vi "Destroy Queues.vi"(8 "error in (no error)":errorcluster) -> (0 "error out":errorcluster)   [LabVIEW 2017]
uses:
  Reference Action.ctl
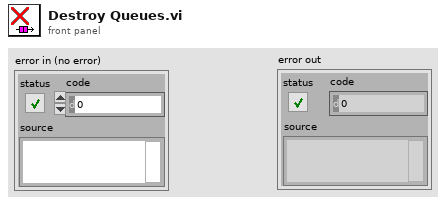
[diagram p1: front panel]
types:
  T1 = typedef "Reference Action.ctl" = enum16{"Set", "Get"}
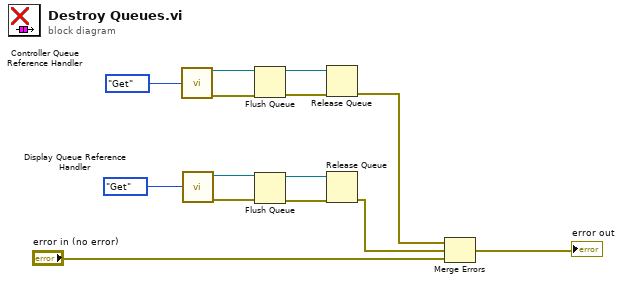
[diagram p0: block diagram]
diagram:
  n1 = call "Controller Queue Reference Handler.vi"("Reference Action"=Reference_Action."Get") -> ("Error Out"=w14:errorcluster, "Queue Ref Out"=w12:refnum<queue>)  [unwired: 9 in]
  n2 = call "Display Queue Reference Handler.vi"("Reference Action"=Reference_Action."Get") -> ("Error Out"=w8:errorcluster, "Queue Ref Out"=w7:refnum<queue>)  [unwired: 9 in]
  n3 = Flush Queue(queue=w12, error in (no error)=w14) -> (queue out=w6:refnum<queue>, error out=w13:errorcluster)  [unwired: 1 out]
  n4 = Flush Queue(queue=w7, error in (no error)=w8) -> (queue out=w5:refnum<queue>, error out=w9:errorcluster)  [unwired: 1 out]
  n5 = Release Queue(queue=w6, error in (no error)=w13) -> (error out=w4:errorcluster)  [unwired: 1 in, 2 out]
  n6 = Release Queue(queue=w5, error in (no error)=w9) -> (error out=w3:errorcluster)  [unwired: 1 in, 2 out]
  n7 = Merge Errors(w4, w3, "error in (no error)") -> (→"error out":errorcluster)
